vi "test error.vi"() -> ()   [LabVIEW 2014]
uses:
  <vilib>/Utility/error.llb/DialogType.ctl
panel:
  out "error?":bool
  out "error out":errorcluster
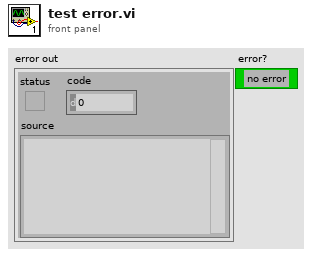
[diagram p1: front panel]
types:
  T1 = typedef "DialogType.ctl" = u16
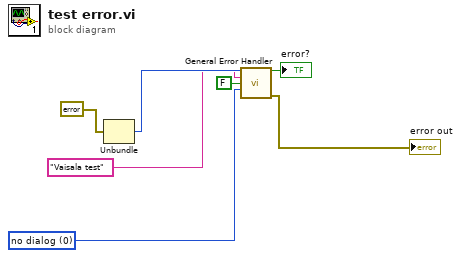
[diagram p0: block diagram]
diagram:
  w4 = T1 0 items=["no dialog", "OK message", "continue or stop message", "OK message + warnings", "continue/stop + warnings"] ("type of dialog (OK msg:1)")
  n1 = Unbundle(errorcluster {"status"=TRUE, "code"=1, "source"="Scan From String (arg 1) in Vaisala Library.lvlib:Vaisala.lvclass:Get Data.vi->DAQ Device.lvlib:Device.lvclass:Actor Core.vi:5880002->Actor Framework.lvlib:Actor.lvclass:Actor.vi:6640012->Actor Framework.lvlib:Actor.lvclass:Actor.vi.ACBRProxyCaller.A9400006"} ("error constant")) -> ("code"=w6:i32)  [unwired: 2 out]
  n2 = call <vilib>:"General Error Handler.vi"("[error code] (0)"=w6, "[error source] (\" \")"="Vaisala test" ("[exception source]"), "search ni.com link visible?(T)"=FALSE, "type of dialog (OK msg:1)"=w4) -> ("error?"=→"error?":bool, "error out"=→"error out":errorcluster)  [unwired: 7 in, 3 out]
